vi "emotion_recognize01.vi"() -> ()   [LabVIEW 2014]
uses:
  <vilib>/sound2/lvsound2.llb/Sampling Mode.ctl
  <vilib>/sound2/lvsound2.llb/Sound Data Format.ctl
  <vilib>/sound2/lvsound2.llb/Sound File Write Open.vi
  <vilib>/sound2/lvsound2.llb/Sound Input Read (DBL).vi
  <vilib>/sound2/lvsound2.llb/Sound File Write (DBL).vi
  <vilib>/sound2/lvsound2.llb/Sound File Info (path).vi
  <vilib>/sound2/lvsound2.llb/Sound File Read Open.vi
  <vilib>/sound2/lvsound2.llb/Sound File Read (DBL).vi
  <vilib>/Utility/file.llb/Write To Spreadsheet File (DBL).vi
  <vilib>/Utility/file.llb/Read From Spreadsheet File (DBL).vi
panel:
  in  "开始":bool
  in  "模型选择":u16(ring) items=["使用内置训练数据", "手动选择训练数据"]
  in  "感情种类":u16(ring) items=["0", "1", "2", "3", "4", "5", "6"]
  in  "训练次数":dbl
  in  "开始训练":T1
  in  "输入数据":path
  in  "特征提取":bool
  in  "启动测试":bool
  in  "结束测试":bool
  in  "path":path=path "D:/sound/1.wav" caption="存储路径"
  in  "录音播放":bool
  in  "循环次数":i32=2
  in  "播放时间":u32=10
  in  "录音时间":u32=10
  out "error out":errorcluster caption="错误输出"
  in  "选项卡控件":enum32{"录音&播放", "特征提取", "训练", "识别"}(tab)
  out "波形图 2":waveform(dbl)[](graph)
  out "?":waveform(dbl)[](graph)
  out "?":string
  out "?":string
  out "结果":string
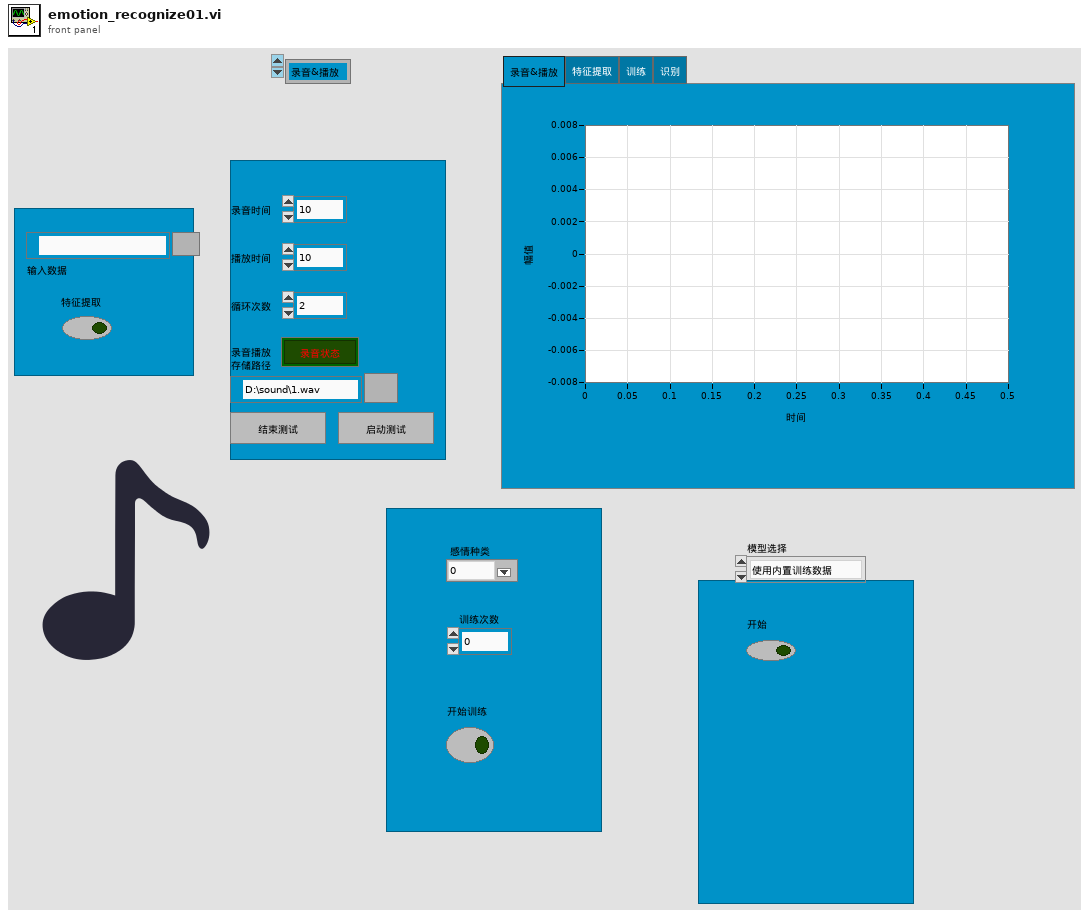
[diagram p1: front panel]
types:
  T1 = typedef "控件 1.ctl" = bool
  T2 = typedef "Sound Data Format.ctl" = cluster{"sample rate (S/s)":dbl, "number of channels":i32, "bits per sample":i32}
  T3 = typedef "Sampling Mode.ctl" = i32
  T4 = typedef "Sound Input Task ID.ctl" = u32
  T5 = typedef "Sound File Refnum.ctl" = refnum<file>
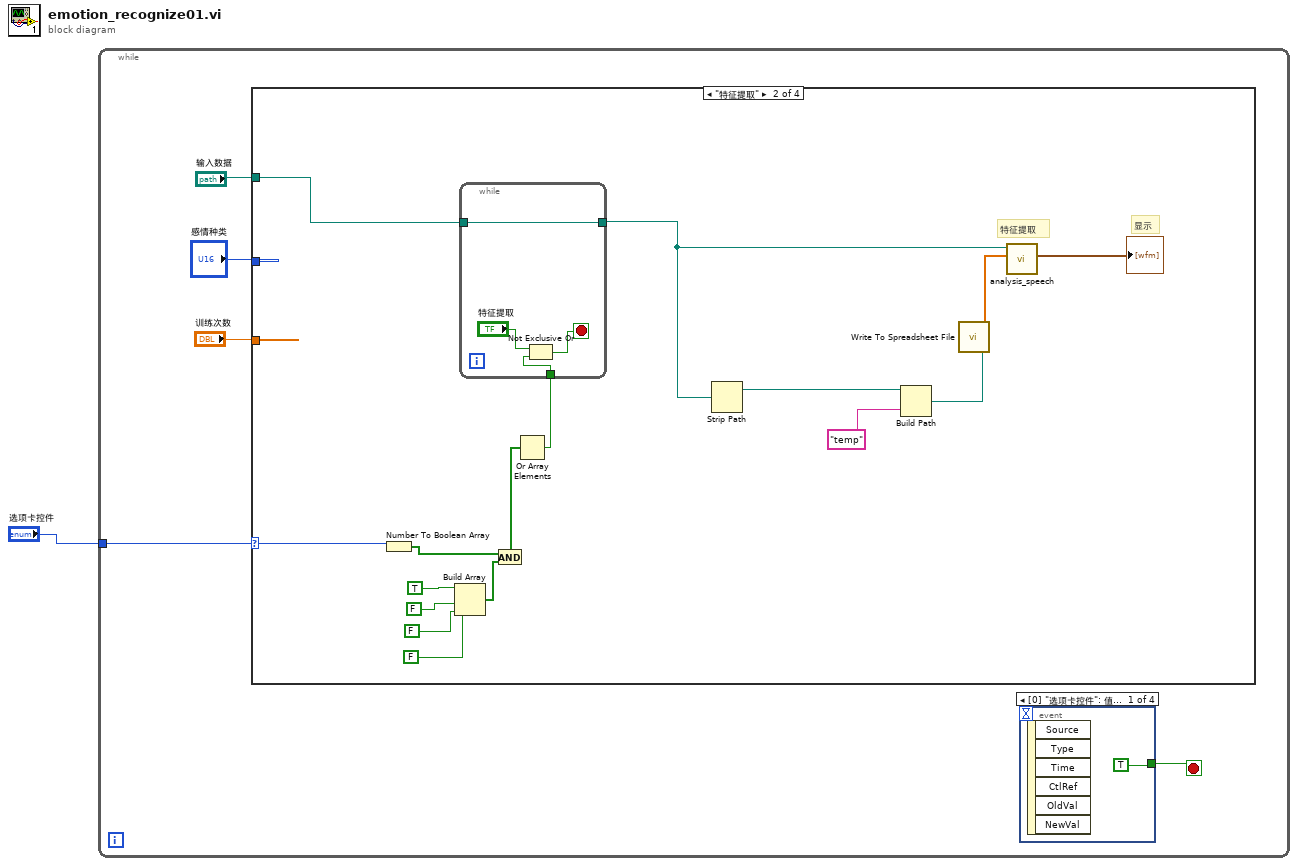
[diagram p0: block diagram]
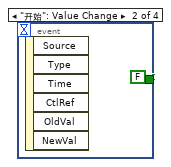
[diagram p2: hidden frame]
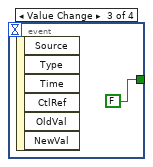
[diagram p3: hidden frame]
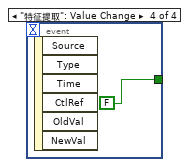
[diagram p4: hidden frame]
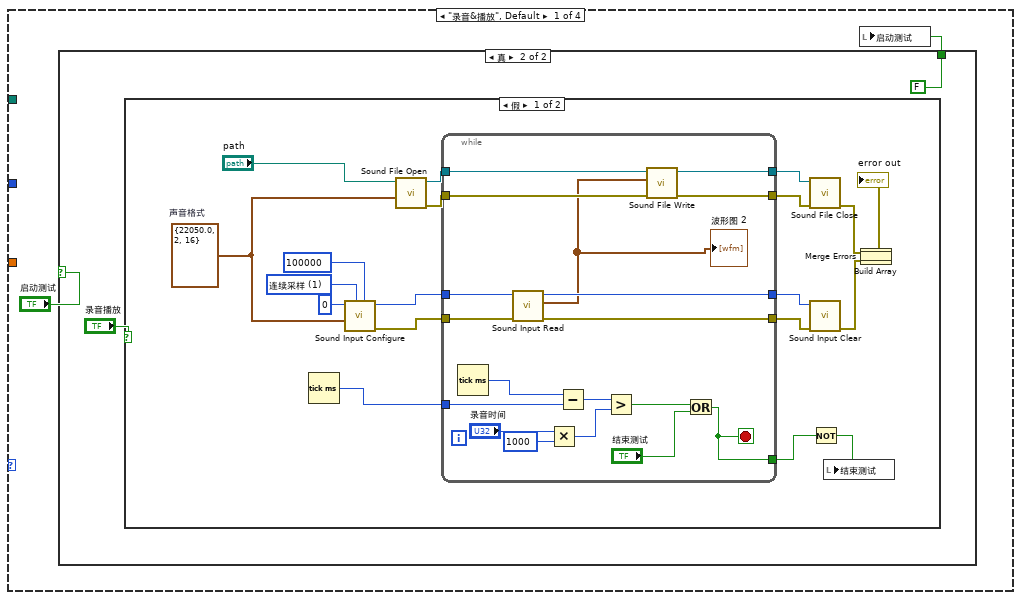
[diagram p5: hidden frame]
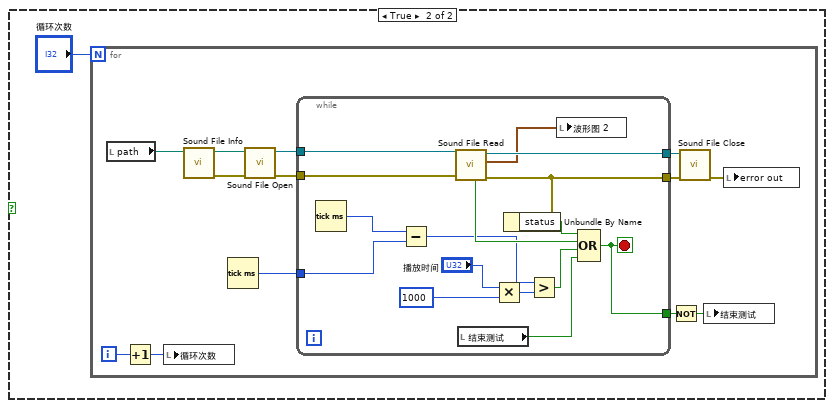
[diagram p7: hidden frame]
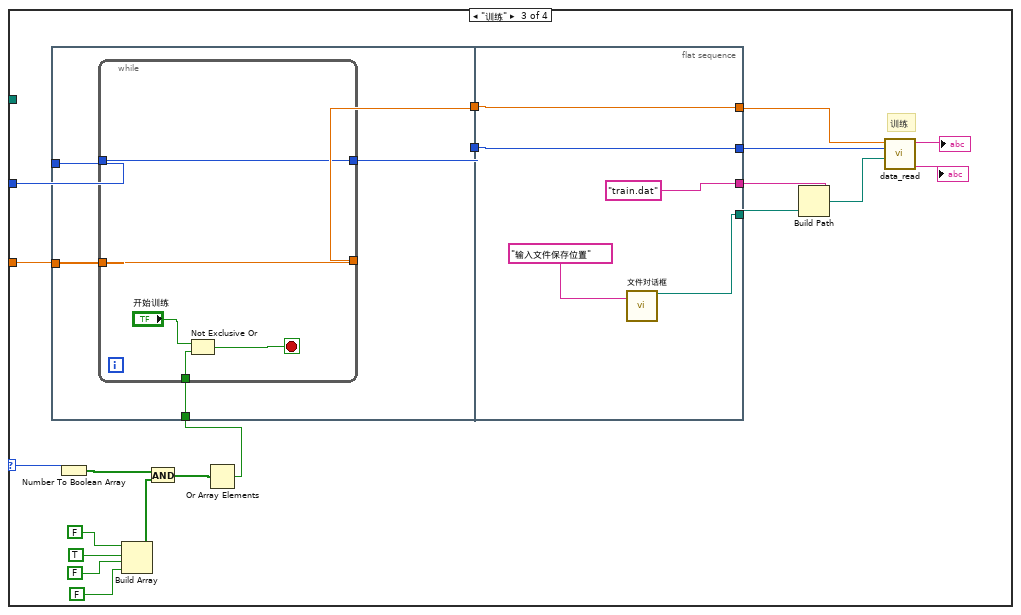
[diagram p8: hidden frame]
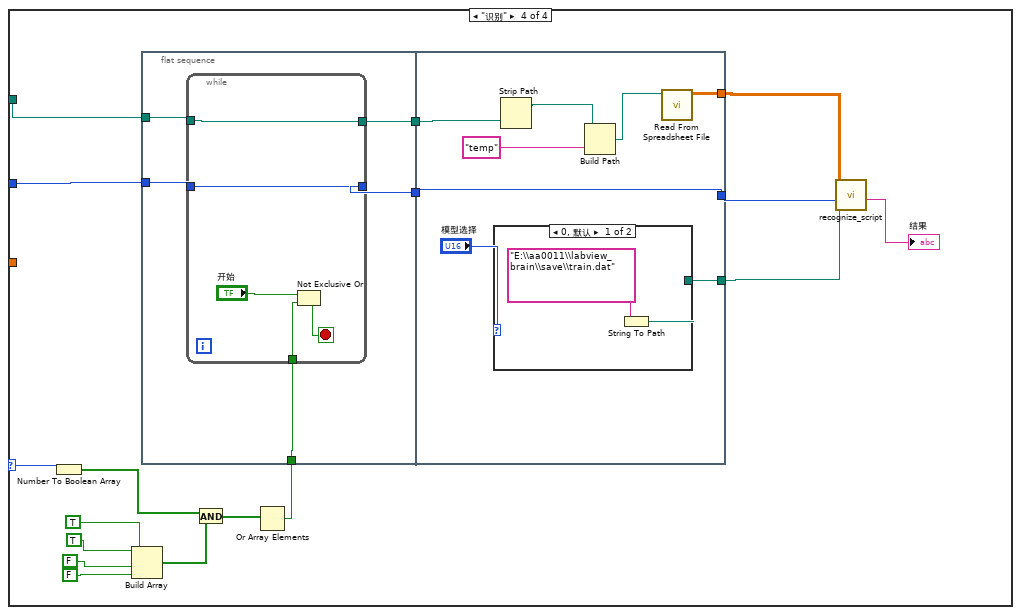
[diagram p9: hidden frame]
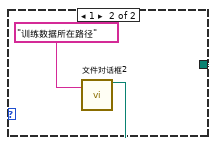
[diagram p10: hidden frame]
diagram:
  n1 = while {
    tunnel: "选项卡控件" -> [w3]
    stop <- w2 stop-if-true
    n2 = case "条件结构" shown="\"特征提取\"" w3 {
      selector: w3 -> [_ w87 w112 w150]
      tunnel: "训练次数" -> [_ _ w120 _]
      tunnel: "感情种类" -> [_ _ w122 w152]
      tunnel: "输入数据" -> [_ w83 _ w154]
      frame "录音&播放", Default {
        n3 = case shown="真" "启动测试" {
          tunnel: [_ FALSE] -> w12
          frame False {
          }
          frame True {
            n4 = case shown="假" "录音播放" {
              frame False {
                w31 = T2 {"sample rate (S/s)"=22050.0, "number of channels"=2, "bits per sample"=16}  # 声音格式
                w32 = T3 1 items=["有限采样", "连续采样"] ("采集模式")
                n5 = Tick Count (ms)() -> (millisecond timer value=w23:u32)
                n6 = call <vilib>:"Sound Input Configure.vi"("number of samples/ch"=100000 ("采集点数"), "sample mode"=w32, "sound format"=w31, "device ID"=u32 0 ("设备号")) -> ("error out"=w28:errorcluster, "task ID"=w29:T4)  [unwired: 1 in, 5 out]
                n7 = call-poly <vilib>:"Sound File Open.vi"("sound format"=w31, "path"="path") -> ("error out"=w21:errorcluster, "sound file refnum"=w27:T5)  [unwired: 1 in, 7 out]
                n8 = while {
                  tunnel: w29 -> [w52]
                  tunnel: w28 -> [w51]
                  tunnel: w27 -> [w50]
                  tunnel: [w49] -> w26
                  tunnel: [w37] -> w25
                  tunnel: [w48] -> w24
                  tunnel: w23 -> [w46]
                  tunnel: [w39] -> w22
                  tunnel: w21 -> [w38]
                  tunnel: [w36] -> w17
                  stop <- w36 stop-if-true
                  n9 = Tick Count (ms)() -> (millisecond timer value=w47:u32)
                  n10 = call-poly <vilib>:"Sound Input Read.vi"("error in (no error)"=w51, "task ID"=w52) -> ("error out"=w37:errorcluster, "data"=w35:waveform(dbl)[], "task ID out"=w49:T4)  [unwired: 2 in, 5 out]
                  "波形图 2" <- w35
                  n11 = Multiply(x="录音时间", y=u32 1000) -> (x*y=w41:u32)
                  n12 = Subtract(x=w47, y=w46) -> (x-y=w45:u32)
                  n13 = Greater?(x=w45, y=w41) -> (0:w43:bool)
                  n14 = call-poly <vilib>:"Sound File Write.vi"("error in (no error)"=w38, "data"=w35, "sound file refnum"=w50) -> ("error out"=w39:errorcluster, "sound file refnum out"=w48:T5)  [unwired: 7 out]
                  n15 = Or(x=w43, y="结束测试") -> (x .or. y?=w36:bool)
                }
                n16 = call <vilib>:"Sound File Close.vi"("error in (no error)"=w22, "sound file refnum"=w24) -> ("error out"=w20:errorcluster)  [unwired: 9 out]
                n17 = call <vilib>:"Sound Input Clear.vi"("error in (no error)"=w25, "task ID"=w26) -> ("error out"=w19:errorcluster)  [unwired: 9 out]
                n18 = Not(x=w17) -> (.not. x?=w16:bool)
                n19 = local write "结束测试"(w16) -> ()
                n20 = Build Array(w20, w19) -> (w15:errorcluster[])
                n21 = Merge Errors(w15) -> (→"error out":errorcluster)
              }
              frame True {
                n22 = for {
                  N: "循环次数" -> [_]
                  i -> [w66]
                  n23 = local read "path"() -> (w64:path)
                  n24 = Increment(x=w66) -> (x+1=w65:i32)
                  n25 = local write "循环次数"(w65) -> ()
                  n26 = call-poly <vilib>:"Sound File Info.vi"("path"=w64) -> ("error out"=w63:errorcluster, "path out"=w62:path)  [unwired: 7 in, 2 out]
                  n27 = Tick Count (ms)() -> (millisecond timer value=w56:u32)
                  n28 = call-poly <vilib>:"Sound File Open.vi"("error in (no error)"=w63, "path"=w62) -> ("error out"=w60:errorcluster, "sound file refnum"=w61:T5)  [unwired: 8 in]
                  n29 = while {
                    tunnel: w61 -> [w82]
                    tunnel: w60 -> [w81]
                    tunnel: [w78] -> w59
                    tunnel: [w80] -> w58
                    tunnel: w56 -> [w76]
                    tunnel: [w71] -> w55
                    stop <- w71 stop-if-true
                    n30 = Tick Count (ms)() -> (millisecond timer value=w77:u32)
                    n31 = Subtract(x=w77, y=w76) -> (x-y=w75:u32)
                    n32 = call-poly <vilib>:"Sound File Read.vi"("error in (no error)"=w81, "sound file refnum"=w82) -> ("error out"=w78:errorcluster, "data"=w67:waveform(dbl)[], "sound file refnum out"=w80:T5, "end of file?"=w79:bool)  [unwired: 5 in, 1 out]
                    n33 = local read "结束测试"() -> (w72:bool)
                    n34 = Multiply(x="播放时间", y=u32 1000) -> (x*y=w70:u32)
                    n35 = Unbundle By Name(w78) -> ("status"=w68:bool)
                    n36 = Greater?(x=w75, y=w70) -> (0:w73:bool)
                    n37 = local write "波形图 2"(w67) -> ()
                    n38 = Compound Arithmetic op=OR(w68, w79, w73, w72) -> (w71:bool)
                  }
                  n39 = Not(x=w55) -> (.not. x?=w54:bool)
                  n40 = call <vilib>:"Sound File Close.vi"("error in (no error)"=w59, "sound file refnum"=w58) -> ("error out"=w57:errorcluster)  [unwired: 9 in]
                  n41 = local write "结束测试"(w54) -> ()
                  n42 = local write "error out"(w57) -> ()
                }
              }
            }
          }
        }
        n43 = local write "启动测试"(w12) -> ()
      }
      frame "特征提取" {
        # "显示"
        # "特征提取"
        n44 = Number To Boolean Array(number=w87) -> (Boolean array=w90:bool[])
        n45 = Build Array(TRUE, FALSE, FALSE, FALSE) -> (w89:bool[])
        n46 = And(x=w90, y=w89) -> (x .and. y?=w88:bool[])
        n47 = Or Array Elements(Boolean array=w88) -> (logical OR=w86:bool)
        n48 = while {
          tunnel: w83 -> [w102]
          tunnel: [w102] -> w94
          tunnel: w86 -> [w100]
          stop <- w99 stop-if-true
          n49 = Not Exclusive Or(1:w100, 2:"特征提取") -> (0:w99:bool)
        }
        n50 = Strip Path(path=w94) -> (stripped path=w97:path)  [unwired: 1 out]
        n51 = Build Path(base path=w97, name or relative path="temp") -> (appended path=w95:path)
        n52 = call "analysis_speech.vi"("文件路径（使用对话框）"=w94) -> ("数组"=w98:dbl[], "波形图表"=→"?":waveform(dbl)[])  [unwired: 9 in]
        n53 = call-poly <vilib>:"Write To Spreadsheet File.vi"("1D data"=w98, "file path (dialog if empty)"=w95) -> ()  [unwired: 6 in, 1 out]
      }
      frame "训练" {
        # "训练"
        n54 = flat-sequence {
          tunnel: w122 -> [w127]
          tunnel: w120 -> [w125]
          tunnel: w111 -> [w123]
          tunnel: [w126] -> w108
          tunnel: [w124] -> w107
          tunnel: [w136] -> w119
          tunnel: [w137] -> w121
          tunnel: w108 -> [w137]
          tunnel: w107 -> [w136]
          tunnel: [w135] -> w106
          tunnel: ["train.dat"] -> w105
          frame #0 {
            n55 = while {
              tunnel: w127 -> [w132]
              tunnel: [w132] -> w126
              tunnel: w125 -> [w131]
              tunnel: [w131] -> w124
              tunnel: w123 -> [w129]
              stop <- w128 stop-if-true
              n56 = Not Exclusive Or(1:w129, 2:"开始训练") -> (0:w128:T1)
            }
          }
          frame #1 {
            n57 = call "文件对话框"("prompt"="输入文件保存位置") -> ("selected path"=w135:path)  [unwired: 11 in, 3 out]
          }
        }
        n58 = Number To Boolean Array(number=w112) -> (Boolean array=w114:bool[])
        n59 = Build Array(FALSE, TRUE, FALSE, FALSE) -> (w113:bool[])
        n60 = And(x=w114, y=w113) -> (x .and. y?=w110:bool[])
        n61 = Or Array Elements(Boolean array=w110) -> (logical OR=w111:bool)
        n62 = Build Path(base path=w106, name or relative path=w105) -> (appended path=w109:path)
        n63 = call "data_read.vi"("路径"=w109, "感情数目"=w121, "训练次数"=w119) -> ("字符串 2"=→"?":string, "字符串"=→"?":string)  [unwired: 6 in, 1 out]
      }
      frame "识别" {
        n64 = Number To Boolean Array(number=w150) -> (Boolean array=w144:bool[])
        n65 = Build Array(TRUE, TRUE, FALSE, FALSE) -> (w143:bool[])
        n66 = flat-sequence {
          tunnel: w154 -> [w159]
          tunnel: w152 -> [w157]
          tunnel: w149 -> [w155]
          tunnel: [w158] -> w141
          tunnel: [w156] -> w140
          tunnel: [w172] -> w151
          tunnel: w141 -> [w171]
          tunnel: w140 -> [w172]
          tunnel: [w167] -> w139
          tunnel: [w165] -> w138
          frame #0 {
            n67 = while {
              tunnel: w159 -> [w164]
              tunnel: [w164] -> w158
              tunnel: w157 -> [w163]
              tunnel: [w163] -> w156
              tunnel: w155 -> [w162]
              stop <- w161 stop-if-true
              n68 = Not Exclusive Or(1:w162, 2:"开始") -> (0:w161:bool)
            }
          }
          frame #1 {
            n69 = case shown="0, 默认" "模型选择" {
              tunnel: [w173 w175] -> w165
              frame 0, Default {
                n70 = String To Path(string="E:\\aa0011\\labview_brain\\save\\train.dat") -> (path=w173:path)
              }
              frame 1 {
                n71 = call "文件对话框2"("prompt"="训练数据所在路径") -> ("selected path"=w175:path)  [unwired: 11 in, 3 out]
              }
            }
            n72 = Strip Path(path=w171) -> (stripped path=w170:path)  [unwired: 1 out]
            n73 = Build Path(base path=w170, name or relative path="temp") -> (appended path=w168:path)
            n74 = call-poly <vilib>:"Read From Spreadsheet File.vi"("file path (dialog if empty)"=w168) -> ("all rows"=w167:dbl[][])  [unwired: 6 in, 4 out]
          }
        }
        n75 = And(x=w144, y=w143) -> (x .and. y?=w142:bool[])
        n76 = Or Array Elements(Boolean array=w142) -> (logical OR=w149:bool)
        n77 = call "recognize_script.vi"("文件路径（使用对话框）"=w138, "数组"=w139, "数值 3"=w151) -> ("结果"=→"结果":string)  [unwired: 6 in, 1 out]
      }
    }
    n78 = event shown="[0] \"选项卡控件\": 值改变" {
      selector: _ -> [_ _ _ _]
      dyn-events: _ -> [_ _ _ _]
      timeout: _ -> [_ _ _ _]
      tunnel: [TRUE FALSE FALSE FALSE] -> w2
      event "选项卡控件": Value Change {
        n79 = event-data() -> ()  [unwired: 1 in, 6 out]
      }
      event "开始": Value Change {
        n80 = event-data() -> ()  [unwired: 1 in, 6 out]
      }
      event Value Change {
        n81 = event-data() -> ()  [unwired: 1 in, 6 out]
      }
      event "特征提取": Value Change {
        n82 = event-data() -> ()  [unwired: 1 in, 6 out]
      }
    }
  }
